vi "Init.vi"(8 "error in (no error)":errorcluster caption="错误输入（无错误）", 11 "UI 输入":refnum<class "UI.lvclass">) -> (0 "error out":errorcluster caption="错误输出", 3 "UI 输出":refnum<class "UI.lvclass">)   [LabVIEW 2019, in "UI.lvlib" / "UI.lvclass"]
uses:
  UI.lvclass
  C:/Program Files (x86)/National Instruments/LabVIEW 2019/vi.lib/ActorFramework/Actor/Actor.lvclass
  ErrorHanlder/ErrorHanlder/ErrorHanlder.lvclass
  Log/Log/Log.lvclass
  UI.lvclass/UI.ctl
  <vilib>/ActorFramework/Message Enqueuer/Message Enqueuer.lvclass/Message Enqueuer.ctl
  <vilib>/ActorFramework/Message Enqueuer/Enqueue.vi
  C:/Program Files (x86)/National Instruments/LabVIEW 2019/vi.lib/ActorFramework/Message/Message.lvclass
  <vilib>/ActorFramework/Message Priority Queue/Priority Enqueue.vi
  <vilib>/ActorFramework/Actor/Actor.lvclass
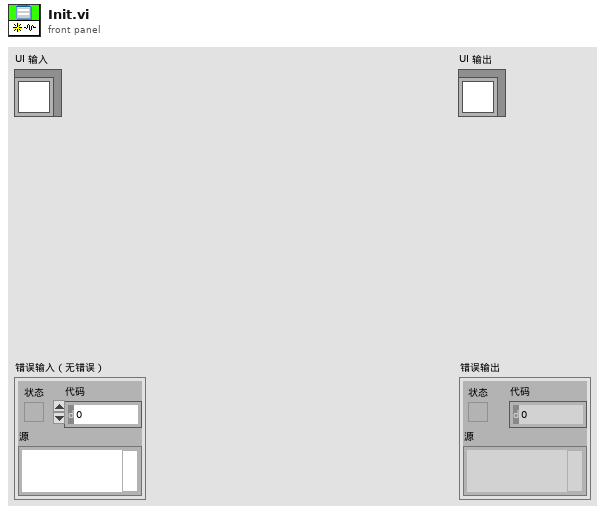
[diagram p1: front panel]
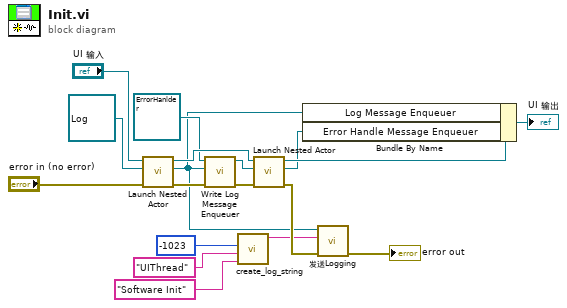
[diagram p0: block diagram]
diagram:
  n1 = call <vilib>:"Launch Nested Actor.vi"("error in (no error)"="error in (no error)", "Nested Actor"=refnum<class "Log.lvclass"> refnum ("Log.lvlib:Log.lvclass"), "Caller Actor in"="UI 输入") -> ("error out"=w10:errorcluster, "Nested Actor's Enqueuer"=w5:refnum<class "Message Enqueuer.lvclass">, "Caller Actor out"=w14:refnum<class "UI.lvclass">)  [unwired: 6 in]
  n2 = call-dynamic "Write Log Message Enqueuer.vi"("error in (no error)"=w10, "操作者框架:消息待入队列"=w5, "ErrorHanlder输入"=refnum<class "ErrorHanlder.lvclass"> refnum ("ErrorHanlder.lvlib:ErrorHanlder.lvclass")) -> ("error out"=w9:errorcluster, "ErrorHanlder输出"=w11:refnum<class "ErrorHanlder.lvclass">)  [unwired: 7 in]
  n3 = call "create_log_string.vi"("source"="Software Init" ("thread"), "thread"="UIThread", "Code"=-1023) -> ("log string"=w4:string)  [unwired: 8 in]
  n4 = call <vilib>:"Launch Nested Actor.vi"("error in (no error)"=w9, "Nested Actor"=w11, "Caller Actor in"=w14) -> ("error out"=w6:errorcluster, "Nested Actor's Enqueuer"=w8:refnum<class "Message Enqueuer.lvclass">, "Caller Actor out"=w18:refnum<class "UI.lvclass">)  [unwired: 6 in]
  n5 = Bundle By Name(cluster=w18, "Log Message Enqueuer"=w5, "Error Handle Message Enqueuer"=w8) -> (→"UI 输出":refnum<class "UI.lvclass">)
  n6 = call "发送Logging.vi"("error in (no error)"=w6, "Log"=w4, "Message Enqueuer"=w5) -> ("error out"=→"error out":errorcluster)  [unwired: 7 in, 1 out]
